vi "Merge Sort 3D Coordinate Arrays.vi"(0 "3D Coordinate Array A":cluster{"x1":dbl, "x2":dbl, "x3":dbl}[](array[cluster]), 1 "Ignore Duplicates? (F)":bool, 3 "3D Cooridnate Array B":cluster{"x1":dbl, "x2":dbl, "x3":dbl}[](array[cluster])) -> (6 "Sorted 3D Coordinate Array":cluster{"x1":dbl, "x2":dbl, "x3":dbl}[](array[cluster]))   [LabVIEW 2013]
panel:
  out "A Index":i32
  out "B Index":i32
  out "B Count":i32
  out "A Count":i32
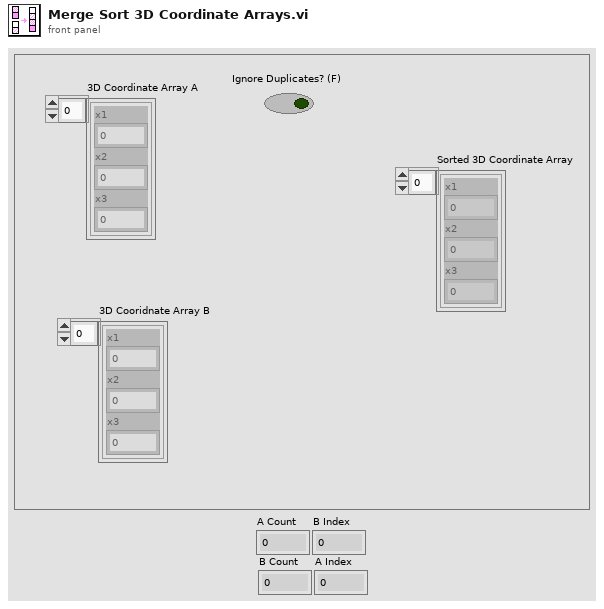
[diagram p1: front panel]
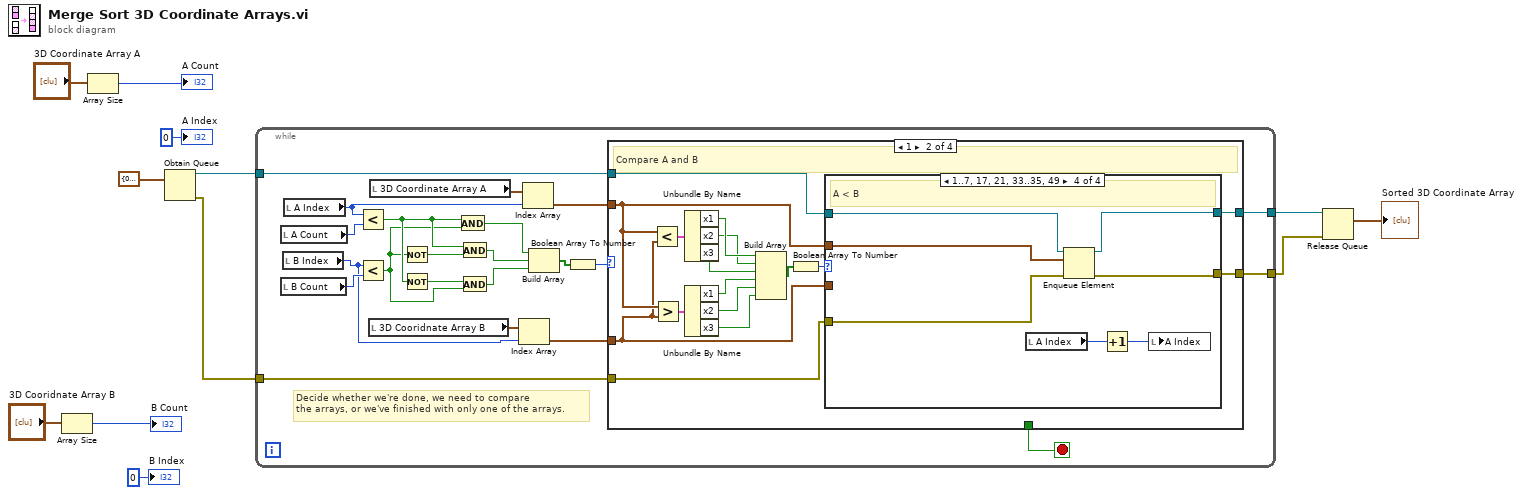
[diagram p0: block diagram]
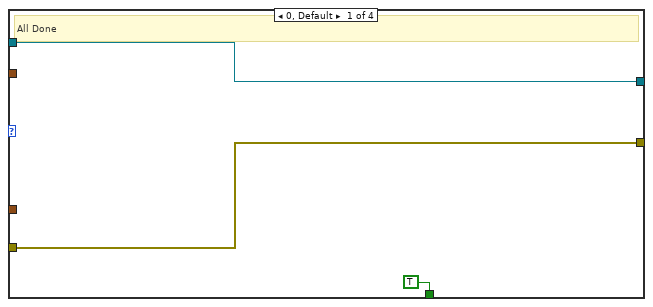
[diagram p2: hidden frame]
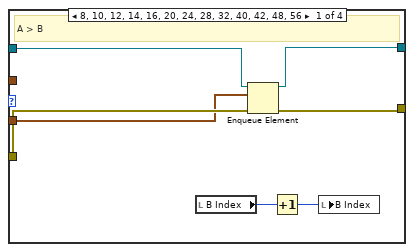
[diagram p3: hidden frame]
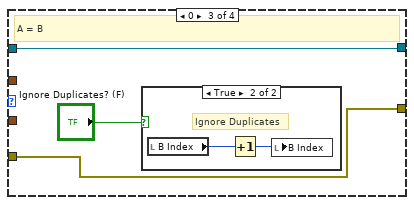
[diagram p5: hidden frame]
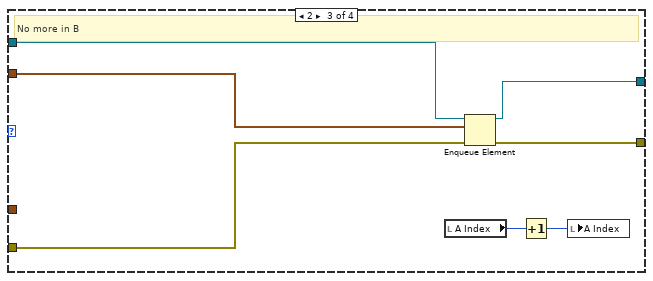
[diagram p7: hidden frame]
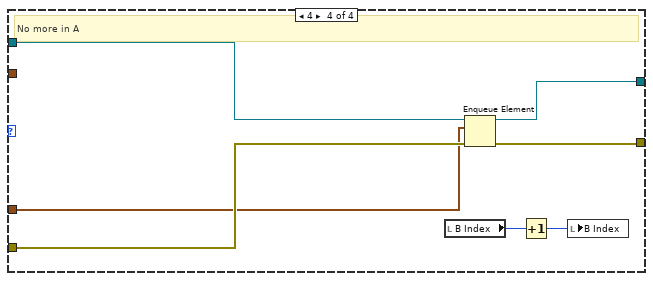
[diagram p8: hidden frame]
diagram:
  n1 = Array Size(array="3D Cooridnate Array B") -> (size(s)=→"B Count":i32)
  n2 = Array Size(array="3D Coordinate Array A") -> (size(s)=→"A Count":i32)
  n3 = Obtain Queue(element data type=cluster{"x1":dbl, "x2":dbl, "x3":dbl} {"x1"=0.0, "x2"=0.0, "x3"=0.0} ("2D Coordinate")) -> (queue out=w11:refnum<queue>, error out=w10:errorcluster)  [unwired: 4 in, 1 out]
  n4 = while {
    tunnel: w11 -> [w23]
    tunnel: [w22] -> w3
    tunnel: [w21] -> w12
    tunnel: w10 -> [w20]
    stop <- w13 stop-if-true
    # "Decide whether we're done, we need to compare\nthe arrays, or we've finished with only one of the arrays."
    n5 = local read "A Count"() -> (w34:i32)
    n6 = local read "B Count"() -> (w33:i32)
    n7 = local read "B Index"() -> (w16:i32)
    n8 = local read "A Index"() -> (w18:i32)
    n9 = Less?(x=w18, y=w34) -> (x < y?=w30:bool)
    n10 = Less?(x=w16, y=w33) -> (x < y?=w29:bool)
    n11 = local read "3D Cooridnate Array B"() -> (w17:cluster{"x1":dbl, "x2":dbl, "x3":dbl}[])
    n12 = local read "3D Coordinate Array A"() -> (w19:cluster{"x1":dbl, "x2":dbl, "x3":dbl}[])
    n13 = Not(x=w29) -> (.not. x?=w27:bool)
    n14 = Not(x=w30) -> (.not. x?=w26:bool)
    n15 = And(x=w30, y=w29) -> (x .and. y?=w32:bool)
    n16 = And(x=w30, y=w27) -> (x .and. y?=w31:bool)
    n17 = And(x=w26, y=w29) -> (x .and. y?=w28:bool)
    n18 = Index Array(array=w17, index=w16) -> (element=w15:cluster{"x1":dbl, "x2":dbl, "x3":dbl})
    n19 = Index Array(array=w19, index=w18) -> (element=w14:cluster{"x1":dbl, "x2":dbl, "x3":dbl})
    n20 = Build Array(w32, w31, w28) -> (w25:bool[])
    n21 = Boolean Array To Number(Boolean array=w25) -> (number=w24:u32)
    n22 = case shown="1" w24 {
      tunnel: w23 -> [w37 w53 w81 w88]
      tunnel: w14 -> [_ w47 w79 _]
      tunnel: w15 -> [_ w46 _ w86]
      tunnel: w20 -> [w36 w48 w80 w87]
      tunnel: [w36 w52 w77 w84] -> w22
      tunnel: [w37 w51 w78 w85] -> w21
      tunnel: [TRUE _ _ _] -> w13
      frame 0, Default {
        # "All Done"
      }
      frame 1 {
        # "Compare A and B"
        n23 = Less?(x=w47, y=w46) -> (x < y?=w45:cluster{"x1":bool, "x2":bool, "x3":bool})
        n24 = Greater?(x=w47, y=w46) -> (0:w44:cluster{"x1":bool, "x2":bool, "x3":bool})
        n25 = Unbundle By Name(w45) -> ("x1"=w43:bool, "x2"=w42:bool, "x3"=w41:bool)
        n26 = Unbundle By Name(w44) -> ("x1"=w40:bool, "x2"=w39:bool, "x3"=w38:bool)
        n27 = Build Array(w43, w42, w41, w40, w39, w38) -> (w50:bool[])
        n28 = Boolean Array To Number(Boolean array=w50) -> (number=w49:u32)
        n29 = case shown="1..7, 17, 21, 33..35, 49" w49 {
          tunnel: w53 -> [w60 w62 w63 w74]
          tunnel: w47 -> [_ _ _ w73]
          tunnel: w46 -> [w54 _ _ _]
          tunnel: w48 -> [w59 w61 w64 w72]
          tunnel: [w57 w61 w64 w70] -> w52
          tunnel: [w58 w62 w63 w71] -> w51
          frame 8, 10, 12, 14, 16, 20, 24, 28, 32, 40, 42, 48, 56 {
            # "A > B"
            n30 = local read "B Index"() -> (w55:i32)
            n31 = Enqueue Element(queue=w60, element=w54, error in (no error)=w59) -> (queue out=w58:refnum<queue>, error out=w57:errorcluster)  [unwired: 1 in, 1 out]
            n32 = Increment(x=w55) -> (x+1=w56:i32)
            n33 = local write "B Index"(w56) -> ()
          }
          frame Default {
            # "Shouldn't happen"
          }
          frame 0 {
            # "A = B"
            n34 = case shown="True" "Ignore Duplicates? (F)" {
              frame False {
              }
              frame True {
                # "Ignore Duplicates"
                n35 = local read "B Index"() -> (w67:i32)
                n36 = Increment(x=w67) -> (x+1=w66:i32)
                n37 = local write "B Index"(w66) -> ()
              }
            }
          }
          frame 1..7, 17, 21, 33..35, 49 {
            # "A < B"
            n38 = local read "A Index"() -> (w68:i32)
            n39 = Enqueue Element(queue=w74, element=w73, error in (no error)=w72) -> (queue out=w71:refnum<queue>, error out=w70:errorcluster)  [unwired: 1 in, 1 out]
            n40 = Increment(x=w68) -> (x+1=w69:i32)
            n41 = local write "A Index"(w69) -> ()
          }
        }
      }
      frame 2 {
        # "No more in B"
        n42 = local read "A Index"() -> (w75:i32)
        n43 = Enqueue Element(queue=w81, element=w79, error in (no error)=w80) -> (queue out=w78:refnum<queue>, error out=w77:errorcluster)  [unwired: 1 in, 1 out]
        n44 = Increment(x=w75) -> (x+1=w76:i32)
        n45 = local write "A Index"(w76) -> ()
      }
      frame 4 {
        # "No more in A"
        n46 = local read "B Index"() -> (w82:i32)
        n47 = Enqueue Element(queue=w88, element=w86, error in (no error)=w87) -> (queue out=w85:refnum<queue>, error out=w84:errorcluster)  [unwired: 1 in, 1 out]
        n48 = Increment(x=w82) -> (x+1=w83:i32)
        n49 = local write "B Index"(w83) -> ()
      }
    }
  }
  n50 = Release Queue(queue=w12, error in (no error)=w3) -> (remaining elements=→"Sorted 3D Coordinate Array":cluster{"x1":dbl, "x2":dbl, "x3":dbl}[])  [unwired: 1 in, 2 out]
  "A Index" <- 0 ("A Index")
  "B Index" <- 0 ("B Index")
